vi "GS1 Factory Reset.vi"() -> ()   [LabVIEW 2017]
uses:
  <vilib>/NI Modbus.llb/MB Serial Master Query Write Single Register (poly).vi
panel:
  out "Error Out":errorcluster
  in  "Tab Control":enum32{"Control Panel", "VISA 1"}(tab)
  in  "VISA resource name":refnum<visa-resource-name>
  in  "Reset to Factory Default":bool
  in  "Stop Loop":bool
  out "VISA resource name out":refnum<visa-resource-name>
  in  "error in":errorcluster
  out "error out":errorcluster
  # "Factory Reset"
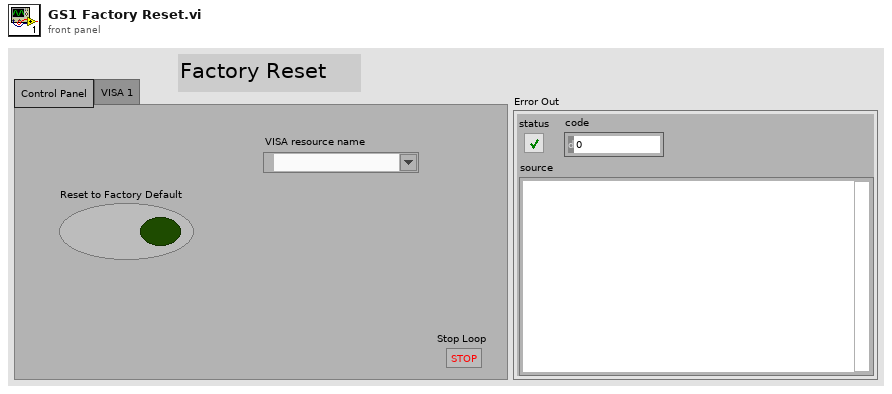
[diagram p1: front panel]
types:
  T1 = cluster{"Mode":enum16{"RTU", "ASCII"}, "Slave Address":u8}
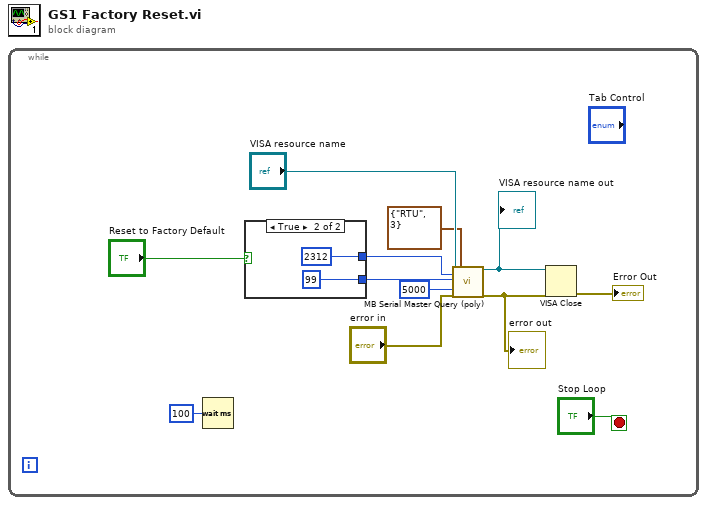
[diagram p0: block diagram]
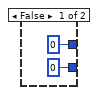
[diagram p2: hidden frame]
diagram:
  n1 = while {
    stop <- "Stop Loop" stop-if-true
    n2 = Wait (ms)(milliseconds to wait=u32 100) -> ()  [unwired: 1 out]
    n3 = case shown="True" "Reset to Factory Default" {
      tunnel: [u16 0 ("Holding Register") u16 99 ("Holding Register")] -> w7
      tunnel: [u16 0 ("Address") u16 2312 ("Address")] -> w6
      frame False {
      }
      frame True {
      }
    }
    n4 = call-poly <vilib>:"MB Serial Master Query (poly).vi"("VISA resource name"="VISA resource name", "Address"=w6, "Holding Register"=w7, "Timeout"=u32 5000, "error in"="error in", "Serial Parameters"=T1 {"Mode"=enum."RTU", "Slave Address"=3}) -> ("VISA resource name out"=w3:refnum<visa-resource-name>, "error out"=w2:errorcluster)  [unwired: 11 in, 1 out]
    "VISA resource name out" <- w3
    "error out" <- w2
    n5 = VISA Close(VISA resource name=w3, error in (no error)=w2) -> (error out=→"Error Out":errorcluster)
  }
